vi "Differences.vi"() -> (0 "XY Graph":cluster{u64[], i64[]}(graph), 3 "WaveForm":i64[](graph), 8 "Last Draw - b[]":i64[](array[numeric]), 11 "Your choices - a[][]":i32[][](array[numeric]))   [LabVIEW 2023]
uses:
  <vilib>/Utility/file.llb/Write Delimited Spreadsheet (I64).vi
panel:
  out "Table Control":string[][](table)
  out "Difference between":i64[][](array[numeric])
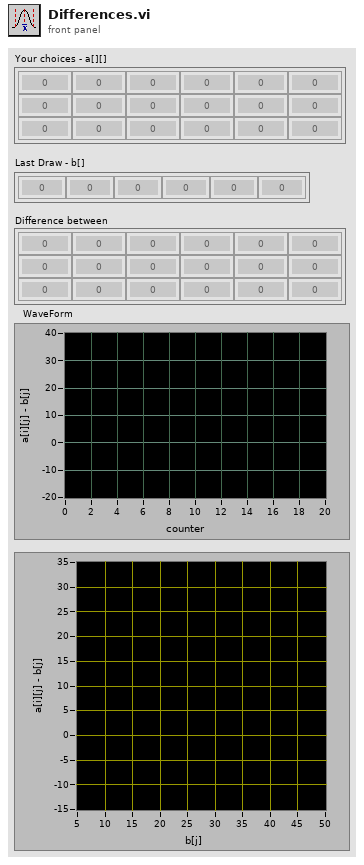
[diagram p1: front panel]
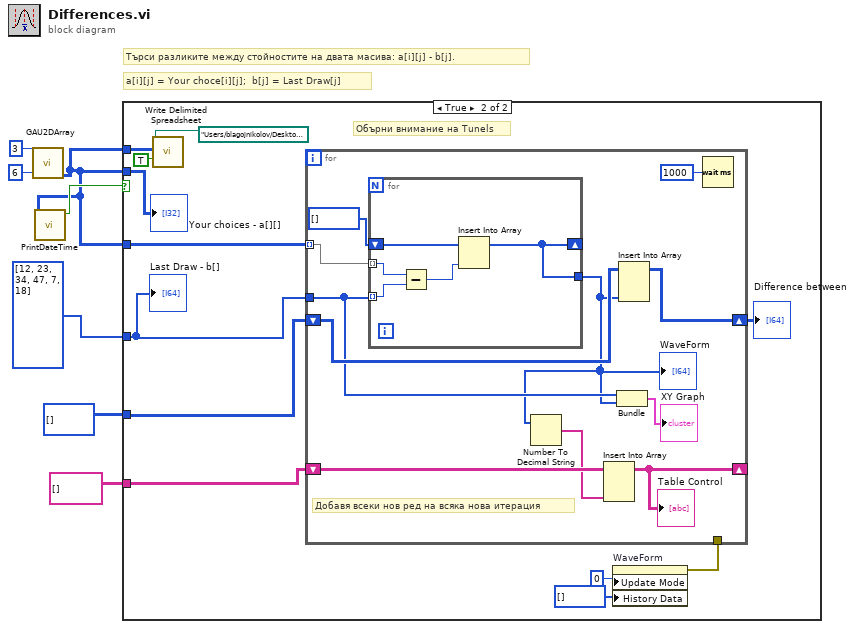
[diagram p0: block diagram]
diagram:
  # "a[i][j] = Your choce[i][j];  b[j] = Last Draw[j]"
  # "Търси разликите между стойностите на двата масива: a[i][j] - b[j]."
  n1 = call "GAU2DArray.vi"("Colums"=6, "Rows"=3) -> ("2D Double Array"=w1:i32[][])  [unwired: 8 in, 1 out]
  n2 = call "PrintDateTime.vi"("2D Double Array"=w1) -> ("T button?"=w2:bool)  [unwired: 10 in]
  n3 = case shown="True" w2 {
    tunnel: i64[][] [] -> [_ w19]
    tunnel: string[][] [] -> [_ w18]
    tunnel: u64[] [12, 23, 34, 47, 7, 18] -> [_ w8]
    tunnel: w1 -> [_ w13]
    tunnel: w1 -> [_ w12]
    tunnel: w1 -> [_ w11]
    frame False {
    }
    frame True {
      # "Обърни внимание на Tunels"
      n4 = call-poly <vilib>:"Write Delimited Spreadsheet.vi"("file path (dialog if empty)"=path "/Users/blagojnikolov/Desktop/@tmp/archive.txt", "2D data"=w11, "append to file? (new file:F)"=TRUE) -> ()  [unwired: 11 in, 2 out]
      n5 = property on="WaveForm" class="WFChart (strict)"("Update Mode"=u8 0, "History Data"=i64[] []) -> (error out=w16:errorcluster)  [unwired: 2 in, 1 out]
      n6 = for {
        tunnel: w13 -> [w30] mode=indexing
        tunnel: w8 -> [w27]
        shift-right: [w21] -> w14
        shift-left: w19 -> [w28]
        shift-right: [w24] -> _
        shift-left: w18 -> [w25]
        tunnel: w16 -> [_]
        # "Добавя всеки нов ред на всяка нова итерация"
        n7 = for {
          tunnel: w27 -> [w34] mode=indexing
          tunnel: w30 -> [w35] mode=indexing
          shift-right: [w31] -> _
          shift-left: i64[] [] -> [w32]
          tunnel: [w31] -> w22
          n8 = Subtract(x=w35, y=w34) -> (x-y=w33:u64)
          n9 = Insert Into Array "Insert Into Array"(array=w32, new element=w33) -> (w31:i64[])  [unwired: 1 in]
        }
        "WaveForm" <- w22
        n10 = Number To Decimal String(number=w22) -> (decimal integer string=w20:string[])  [unwired: 1 in]
        n11 = Insert Into Array "Insert Into Array"(array=w25, new element=w20) -> (w24:string[][])  [unwired: 2 in]
        "Table Control" <- w24
        n12 = Bundle(w27, w22) -> (→"XY Graph":cluster{u64[], i64[]})  [unwired: 1 in]
        n13 = Insert Into Array "Insert Into Array"(array=w28, new element=w22) -> (w21:i64[][])  [unwired: 2 in]
        n14 = Wait (ms)(milliseconds to wait=u32 1000) -> ()  [unwired: 1 out]
      }
      "Difference between" <- w14
      "Your choices - a[][]" <- w12
      "Last Draw - b[]" <- w8
    }
  }
